vi "get_array_from_json_safe.vi"(11 "<JSON>输入":string) -> (3 "<JSON>输出":string[](array[string]))   [LabVIEW 2020]
uses:
  <vilib>/JDP Science/JSONtext/Next JSON Value.vi
  <vilib>/JDP Science/JSONtext/String Subset.vi
  <vilib>/JDP Science/JSONtext/Parsing/Advance past next JSON Value (inlined COPY).vi
  <vilib>/JDP Science/JSONtext/Parsing/Advance past whitespace.vi
  <vilib>/JDP Science/JSONtext/Parsing/Advance past String.vi
  <vilib>/JDP Science/JSONtext/Parsing/Advance past Number.vi
  <vilib>/JDP Science/JSONtext/Parsing/Advance past Line Ending.vi
  <vilib>/JDP Science/JSONtext/Parsing/Parse Full Path or Item Name.vi
  <vilib>/JDP Science/JSONtext/Parsing/Advance past Array.vi
  <vilib>/JDP Science/JSONtext/Parsing/Advance past Object.vi
  <vilib>/JDP Science/JSONtext/support/Error Cluster From Code.vi
  <vilib>/JDP Science/JSONtext/Offset/Find Item Locations by Path.vi
  <vilib>/JDP Science/JSONtext/JSONtext.lvlib
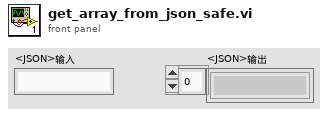
[diagram p1: front panel]
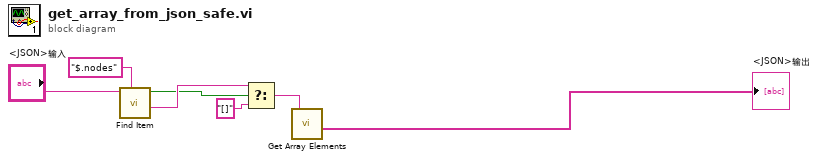
[diagram p0: block diagram]
diagram:
  n1 = call <vilib>:"Find Item.vi"("$Path or Item Name"="$.nodes", "JSON"="<JSON>输入") -> ("<JSON>"=w5:string, "Found"=w4:bool)  [unwired: 6 in, 2 out]
  n2 = Select(t=w5, s=w4, f="[]") -> (s? t:f=w7:string)
  n3 = call <vilib>:"Get Array Elements.vi"("JSON"=w7) -> ("<JSON>"=→"<JSON>输出":string[])  [unwired: 8 in, 2 out]
